vi "ReadCurrent.vi"(8 "error in (no error)":errorcluster, 11 "reference in":refnum<class "VdKeySightMM-A1.lvclass">) -> (0 "error out":errorcluster, 2 "Current":dbl, 3 "reference out":refnum<class "VdKeySightMM-A1.lvclass">)   [LabVIEW 2020, in "MulitMeters.lvlib" / "VdKeySightMM-A1.lvclass"]
uses:
  VdKeySightMM-A1.lvclass
  VdTcpIP_class/VdTcpIP.lvclass
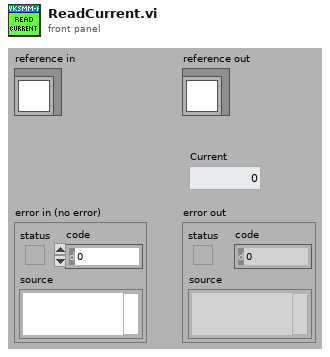
[diagram p1: front panel]
types:
  T1 = typedef "MulitMeters.lvlib/VdKeySightMM-A1.lvclass/ObjectAttributes.ctl" = cluster{"VdTcpIP":refnum<class "VdTcpIP.lvclass">}
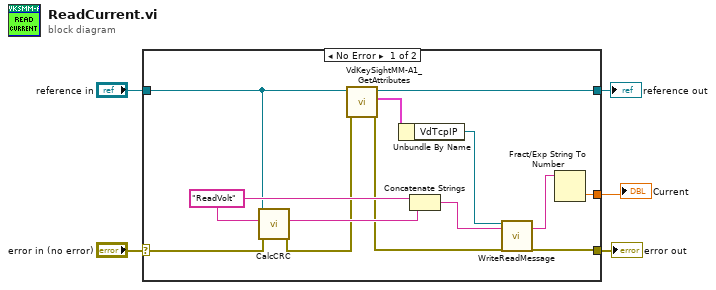
[diagram p0: block diagram]
diagram:
  n1 = case shown="No Error" "error in (no error)" {
    selector: "error in (no error)" -> [w7 w20]
    tunnel: [w11 w20] -> w4
    tunnel: [w17 w19] -> w2
    tunnel: "reference in" -> [w8 w19]
    tunnel: [w9 _] -> w1
    frame No Error {
      w14 = "ReadVolt"
      n2 = call-dynamic "CalcCRC.vi"("error in (no error)"=w7, "TextIn"=w14, "reference in"=w8) -> ("error out"=w6:errorcluster, "CrcOut"=w13:string)  [unwired: 6 in, 1 out]
      n3 = call "VdKeySightMM-A1_GetAttributes.vi"("error in (no error)"=w6, "reference in"=w8) -> ("error out"=w12:errorcluster, "Data"=w18:T1, "reference out"=w17:refnum<class "VdKeySightMM-A1.lvclass">)  [unwired: 6 in, 1 out]
      n4 = Unbundle By Name(w18) -> ("VdTcpIP"=w16:refnum<class "VdTcpIP.lvclass">)
      n5 = Concatenate Strings(w14, w13) -> (w15:string)
      n6 = call "WriteReadMessage.vi"("reference"=w16, "MessageToWrite"=w15, "error in (no error)"=w12) -> ("ReturnedMessage"=w10:string, "error out"=w11:errorcluster)  [unwired: 13 in, 2 out]
      n7 = Fract/Exp String To Number(string=w10) -> (number=w9:dbl)  [unwired: 3 in, 1 out]
    }
    frame Error {
    }
  }
  "error out" <- w4
  "reference out" <- w2
  "Current" <- w1
